vi "Curtin1_NewLine.vi"(9 "origin in":cluster{"x":i16, "y":i16}, 10 "text rect":T1, 11 "Bounds":T2) -> (3 "origin out":cluster{"x":i16, "y":i16})   [LabVIEW 2022 SP3]
uses:
  <vilib>/Utility/miscctls.llb/LVBoundsTypeDef.ctl
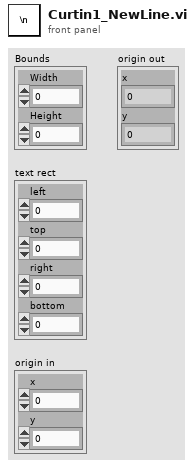
[diagram p1: front panel]
types:
  T1 = cluster{"left":i16, "top":i16, "right":i16, "bottom":i16}
  T2 = typedef "LVBoundsTypeDef.ctl" = cluster{"Width":u32, "Height":u32}
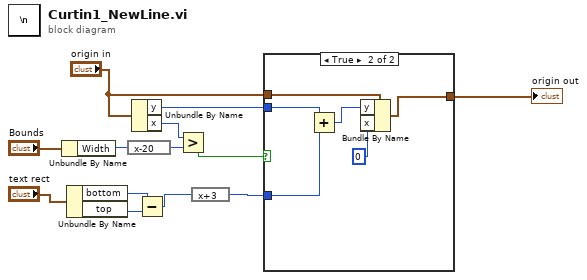
[diagram p0: block diagram]
diagram:
  n1 = Unbundle By Name("Bounds") -> ("Width"=w11:u32)
  n2 = Unbundle By Name("text rect") -> ("bottom"=w2:i16, "top"=w3:i16)
  n3 = expression code="x-20"(w11) -> (w13:u32)
  n4 = Unbundle By Name("origin in") -> ("y"=w5:i16, "x"=w9:i16)
  n5 = Subtract(x=w2, y=w3) -> (x-y=w1:i16)
  n6 = Greater?(x=w9, y=w13) -> (0:w8:bool)
  n7 = expression code="x+3"(w1) -> (w4:i16)
  n8 = case shown="True" w8 {
    tunnel: "origin in" -> [w14 w20]
    tunnel: [w14 w19] -> w6
    tunnel: w5 -> [_ w17]
    tunnel: w4 -> [_ w16]
    frame False {
    }
    frame True {
      n9 = Add(x=w17, y=w16) -> (x+y=w18:i16)
      n10 = Bundle By Name(cluster=w20, "y"=w18, "x"=i16 0 ("y")) -> (w19:cluster{"x":i16, "y":i16})
    }
  }
  "origin out" <- w6
